vi "Online_Statistic_Measurement.vi"(8 "error in (no error)":errorcluster, 10 "New_Measurement":dbl, 11 "Online_Statistic in":refnum<class "Online_Statistic.lvclass">) -> (0 "error out":errorcluster, 3 "Online_Statistic out":refnum<class "Online_Statistic.lvclass">)   [LabVIEW 2021, in "Online_Statistic.lvclass"]
uses:
  Online_Statistic.lvclass
  Online_Statistic.lvclass/Online_Statistic.ctl
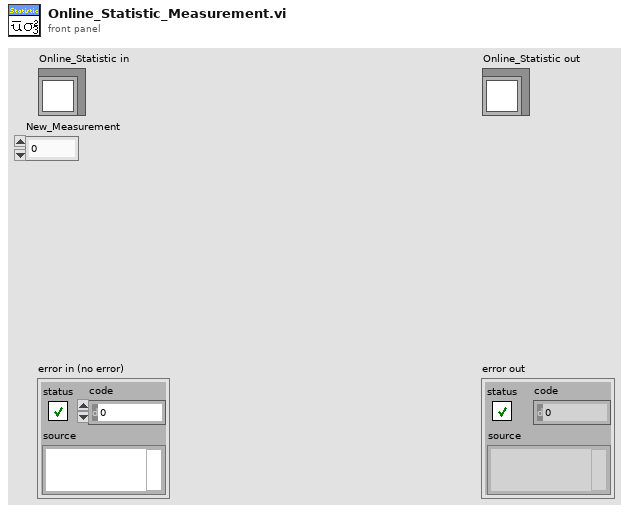
[diagram p1: front panel]
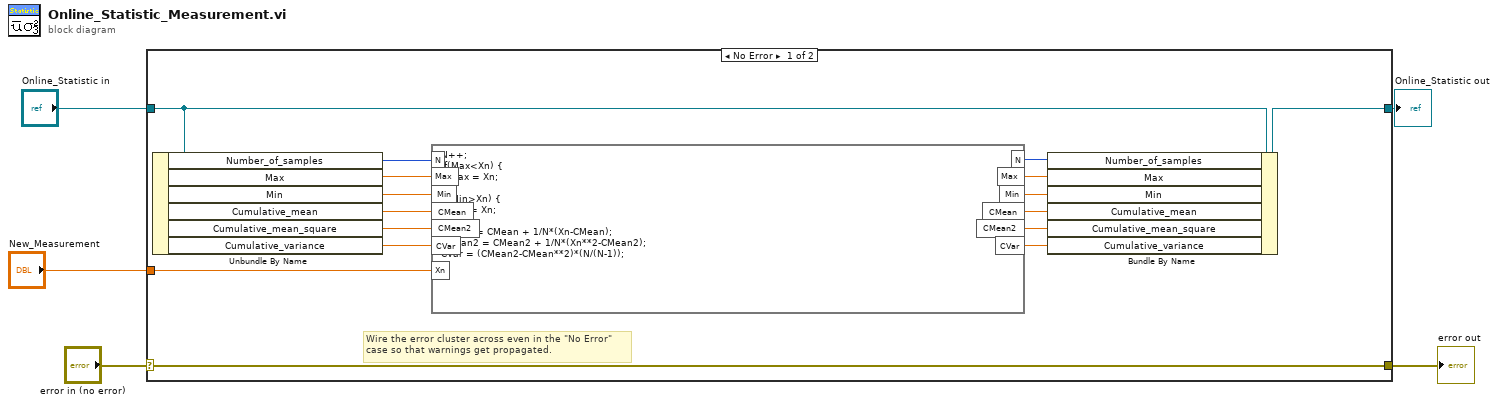
[diagram p0: block diagram]
diagram:
  n1 = case shown="No Error" "error in (no error)" {
    selector: "error in (no error)" -> [w21 w23]
    tunnel: [w21 w23] -> w4
    tunnel: [w6 w22] -> w2
    tunnel: "Online_Statistic in" -> [w7 w22]
    tunnel: "New_Measurement" -> [w14 _]
    frame No Error {
      # "Wire the error cluster across even in the \"No Error\"\ncase so that warnings get propagated."
      n2 = Unbundle By Name(w7) -> ("Number_of_samples"=w20:i32, "Max"=w19:dbl, "Min"=w18:dbl, "Cumulative_mean"=w17:dbl, "Cumulative_mean_square"=w16:dbl, "Cumulative_variance"=w15:dbl)
      n3 = formula code="N++;\nif(Max<Xn) {\n   Max = Xn; \n}\nif(Min>Xn) {\n   Min = Xn; \n}\nCMean = CMean + 1/N*(Xn-CMean);\nCMean2 = CMean2 + 1/N*(Xn**2-CMean2);\nCVar = (CMean2-CMean**2)*(N/(N-1));"("N"=w20, "Max"=w19, "Min"=w18, "CMean"=w17, "CMean2"=w16, "CVar"=w15, "Xn"=w14) -> ("N"=w13:i32, "Max"=w12:dbl, "Min"=w11:dbl, "CMean"=w10:dbl, "CMean2"=w9:dbl, "CVar"=w8:dbl)
      n4 = Bundle By Name(cluster=w7, "Number_of_samples"=w13, "Max"=w12, "Min"=w11, "Cumulative_mean"=w10, "Cumulative_mean_square"=w9, "Cumulative_variance"=w8) -> (w6:refnum<class "Online_Statistic.lvclass">)
    }
    frame Error {
    }
  }
  "error out" <- w4
  "Online_Statistic out" <- w2
